vi "ActivateToggleControls (SubVI).vi"(0 "Left refnum":refnum<vi>, 1 "Current stage position [mm]":cluster{"X":dbl, "Y":dbl, "Z":dbl}, 5 "Right refnum":refnum<vi>, 7 "Forward refnum":refnum<vi>, 9 "Backward refnum":refnum<vi>, 11 "error in (no error)":errorcluster, 12 "Jog step size":T1, 13 "Up refnum":refnum<vi>, 14 "Down refnum":refnum<vi>) -> (15 "error out":errorcluster)   [LabVIEW 2017]
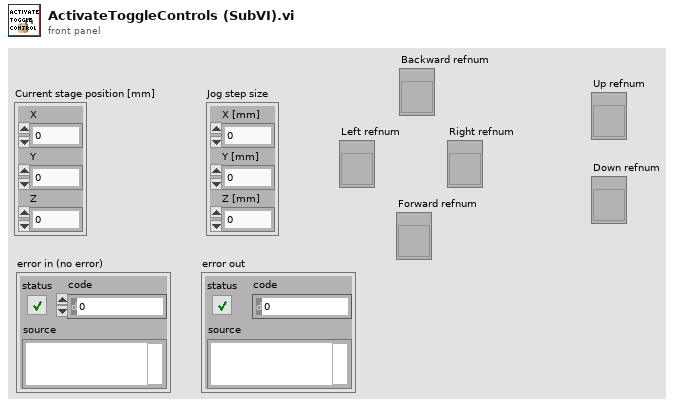
[diagram p1: front panel]
types:
  T1 = cluster{"X [mm]":dbl, "Y [mm]":dbl, "Z [mm]":dbl}
  T2 = enum8{"Enabled", "Disabled", "Disabled and Grayed Out"}
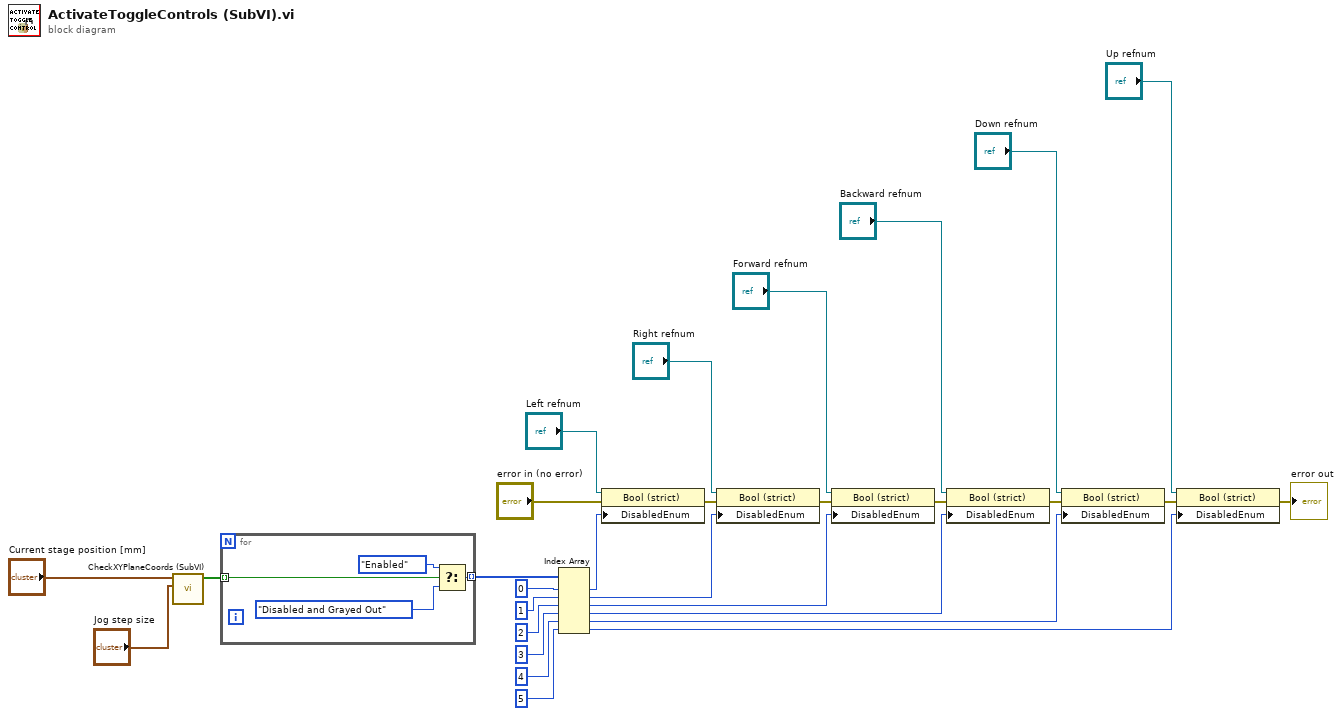
[diagram p0: block diagram]
diagram:
  n1 = call "CheckXYPlaneCoords (SubVI).vi"("Jog Distance"="Jog step size", "Go to Coordinates"="Current stage position [mm]") -> ("Pass record"=w14:bool[])  [unwired: 9 in]
  n2 = for {
    tunnel: w14 -> [w33] mode=indexing
    tunnel: [w30] -> w15 mode=indexing
    n3 = Select(t=T2."Enabled" ("Disabled"), s=w33, f=T2."Disabled and Grayed Out" ("Disabled")) -> (s? t:f=w30:T2)
  }
  n4 = Index Array(array=w15, index #1=0 ("index"), index #2=1 ("index"), index #3=2 ("index"), index #4=3 ("index"), index #5=4 ("index"), index #6=5 ("index")) -> (element #1=w20:T2, element #2=w21:T2, element #3=w23:T2, element #4=w25:T2, element #5=w2:T2, element #6=w1:T2)
  n5 = property on="Property Node" class="Bool (strict)"(reference="Left refnum", error in="error in (no error)", "DisabledEnum"=w20) -> (error out=w22:errorcluster)  [unwired: 1 out]
  n6 = property on="Property Node" class="Bool (strict)"(reference="Right refnum", error in=w22, "DisabledEnum"=w21) -> (error out=w24:errorcluster)  [unwired: 1 out]
  n7 = property on="Property Node" class="Bool (strict)"(reference="Forward refnum", error in=w24, "DisabledEnum"=w23) -> (error out=w26:errorcluster)  [unwired: 1 out]
  n8 = property on="Property Node" class="Bool (strict)"(reference="Backward refnum", error in=w26, "DisabledEnum"=w25) -> (error out=w8:errorcluster)  [unwired: 1 out]
  n9 = property on="Property Node" class="Bool (strict)"(reference="Down refnum", error in=w8, "DisabledEnum"=w2) -> (error out=w6:errorcluster)  [unwired: 1 out]
  n10 = property on="Property Node" class="Bool (strict)"(reference="Up refnum", error in=w6, "DisabledEnum"=w1) -> (error out=→"error out":errorcluster)  [unwired: 1 out]
